vi "motor_control_voltage.vi"(8 "Error In":errorcluster, 10 "Numeric":dbl, 11 "Physical Channel":tag) -> (0 "error out":errorcluster)   [LabVIEW 2013]
uses:
  <vilib>/DAQmx/write.llb/DAQmx Write (Analog DBL 1Chan 1Samp).vi
  <vilib>/DAQmx/create/channels.llb/DAQmx Create Channel (AO-Voltage-Basic).vi
  <vilib>/DAQmx/miscellaneous.llb/DAQmx Fill In Error Info.vi
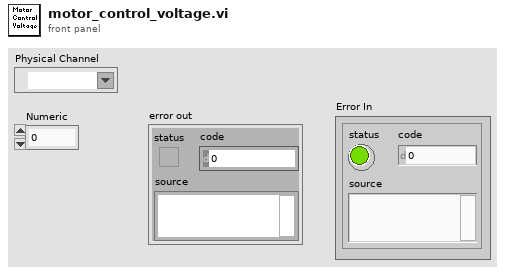
[diagram p1: front panel]
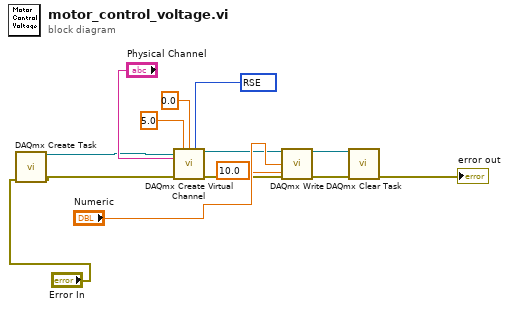
[diagram p0: block diagram]
diagram:
  w1 = 10083 items=["Default"=-1, "RSE"=10083, "Differential"=10106, "Pseudodifferential"=12529] ("output terminal configuration")
  n1 = call <vilib>:"DAQmx Create Task.vi"("error in"="Error In") -> ("task out"=w4:refnum<k21>, "error out"=w2:errorcluster)  [unwired: 13 in]
  n2 = call-poly <vilib>:"DAQmx Create Virtual Channel.vi"("task in"=w4, "maximum value"=5.0, "minimum value"=0.0 ("maximum value"), "output terminal configuration"=w1, "physical channels"="Physical Channel", "error in"=w2) -> ("task out"=w7:refnum<k21>, "error out"=w6:errorcluster)  [unwired: 8 in]
  n3 = call-poly <vilib>:"DAQmx Write.vi"("task/channels in"=w7, "data"="Numeric", "timeout"=10.0, "error in"=w6) -> ("task out"=w10:refnum<k21>, "error out"=w9:errorcluster)  [unwired: 9 in, 1 out]
  n4 = call <vilib>:"DAQmx Clear Task.vi"("task in"=w10, "error in"=w9) -> ("error out"=→"error out":errorcluster)  [unwired: 13 in]
